vi "VgSweep_Bdep.vi"(8 "Start sweeping":bool) -> ()   [LabVIEW 2015]
uses:
  <vilib>/Utility/file.llb/Read From Spreadsheet File (DBL).vi
panel:
  in  "B-table String":string
  in  "Time Stamp":timestamp
  in  "Stabilisation (min)":dbl=0.8 max=4.0 step=1.0
  in  "Custom Folder":string
  out "Communication":string
  in  "Step (T)":dbl=12.0 min=-4.0 max=4.0 step=0.1 format="%.3f"
  out "Experiment ends at:":string
  out "B Array":dbl[](array[numeric])
  in  "Faster":dbl=10.0
  in  "HigherRateBack?":bool
  out "Hours":dbl format="%.1f"
  out "Estimated time of experiment:":i16
  out "# of connections":i16=1 min=-4 max=4 step=1
  in  "Final B (T)":dbl=12.0 min=-4.0 max=4.0 step=0.1 format="%.3f"
  in  "Initial B (T)":dbl min=-4.0 max=4.0 step=0.1 format="%.3f"
  in  "V2:":dbl=1.0 min=-4.0 max=4.0 step=0.1 format="%.3f"
  in  "Sweep rate , V/min":dbl=0.6 min=0.0 max=1.0 step=0.01 format="%.4f"
  in  "V1:":dbl min=-4.0 max=4.0 step=0.1 format="%.3f"
  # "Define interval of gate voltage\nfor main Keithley 2400 (address 12):"
  # "Copy and paste  the \nvalues of B field here.\nIf this string is empty \nthe table is filled \nautomatically."
  # "Set temperatures at which sweeps\nare made"
  # "Go to Initial T?"
  # "min."
  # "="
  # "hours"
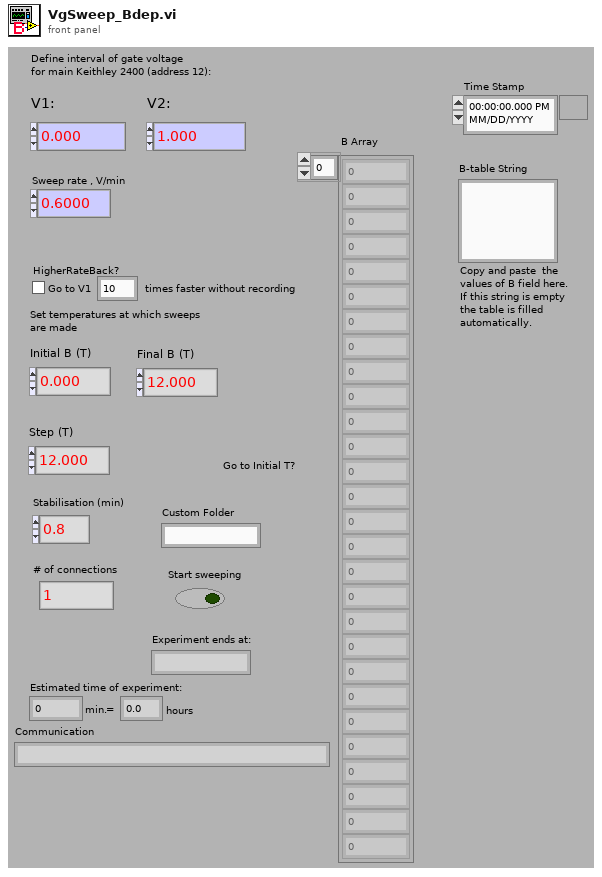
[diagram p1: front panel]
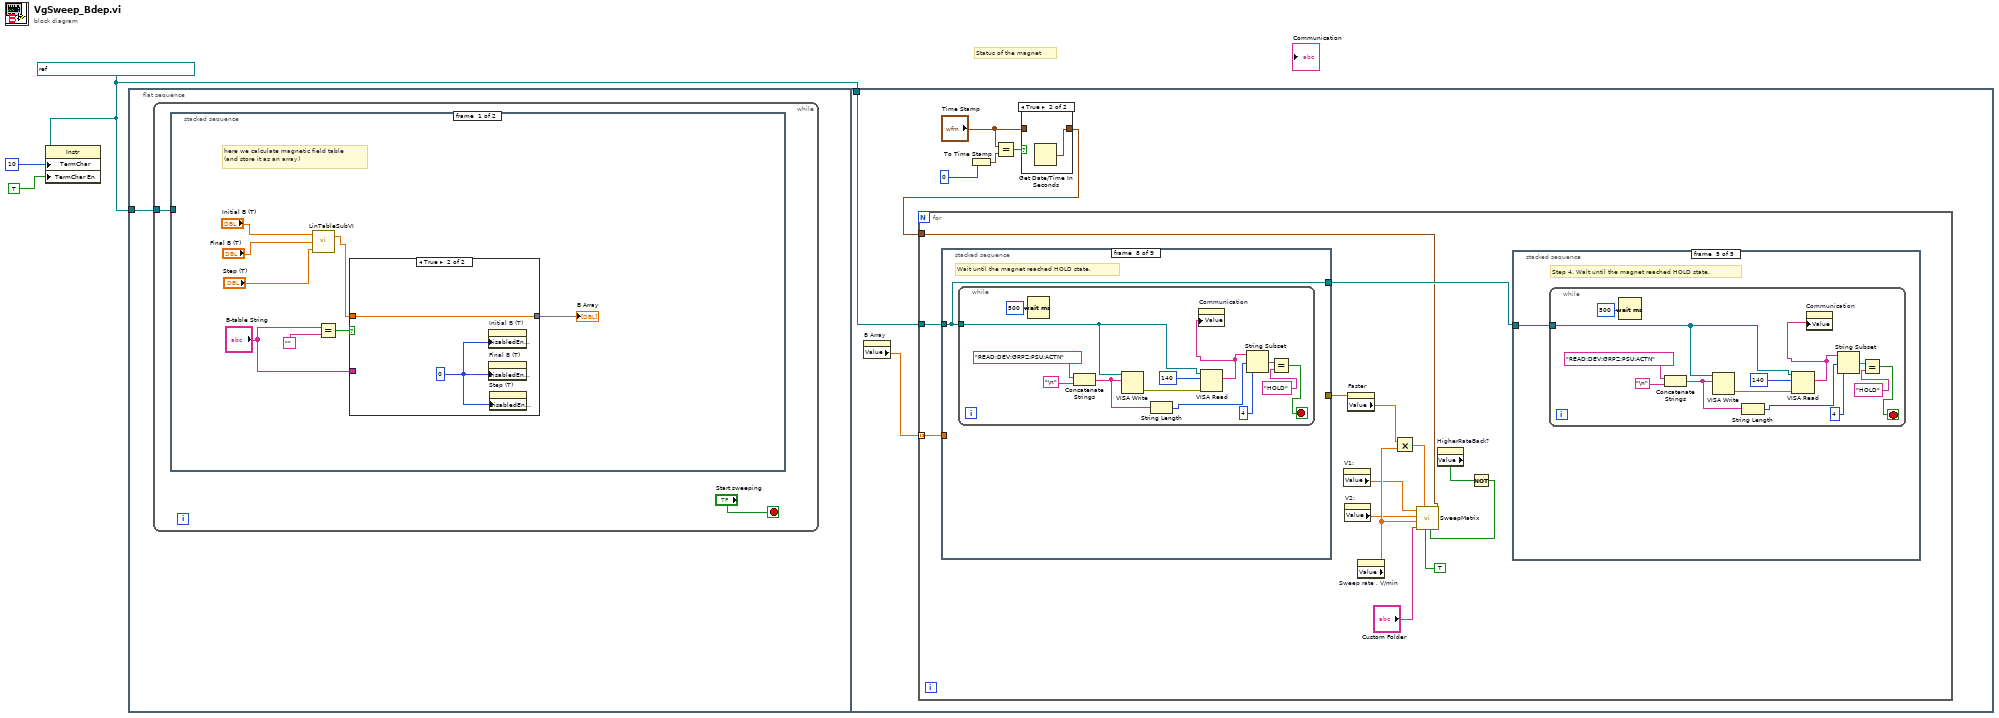
[diagram p0: block diagram]
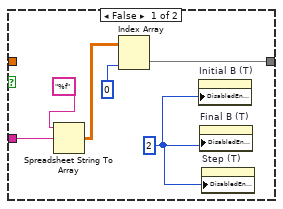
[diagram p2: hidden frame]
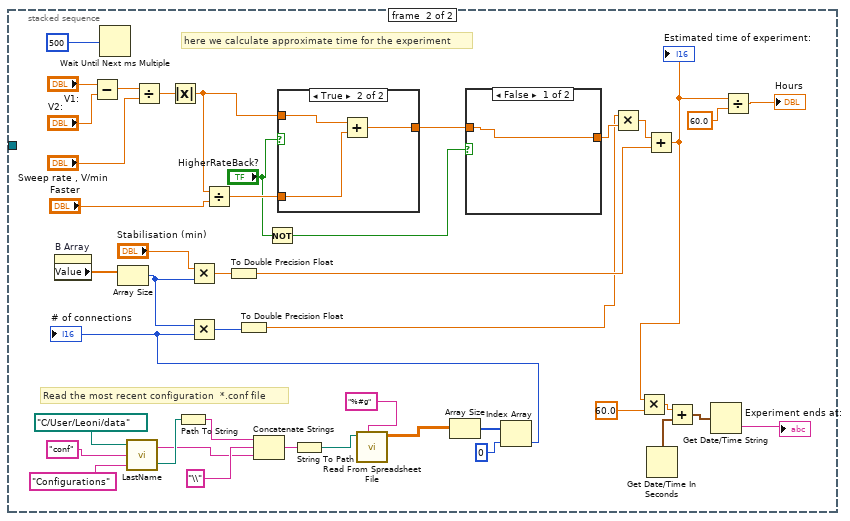
[diagram p3: hidden frame]
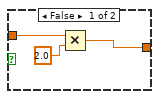
[diagram p4: hidden frame]
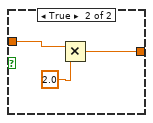
[diagram p5: hidden frame]
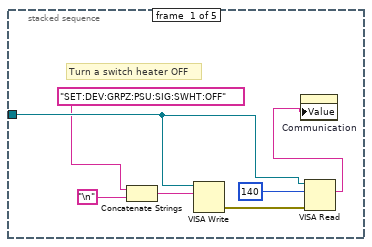
[diagram p7: hidden frame]
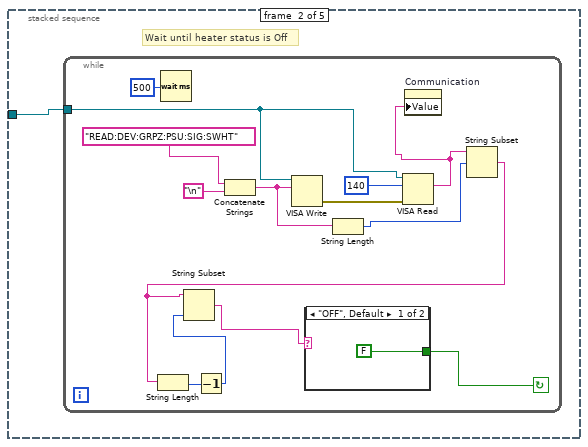
[diagram p8: hidden frame]
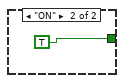
[diagram p9: hidden frame]
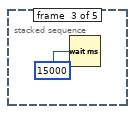
[diagram p10: hidden frame]
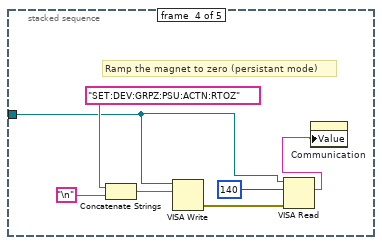
[diagram p11: hidden frame]
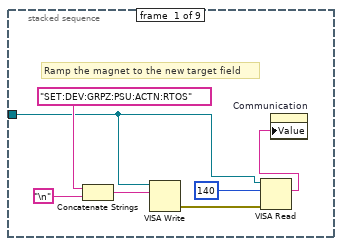
[diagram p12: hidden frame]
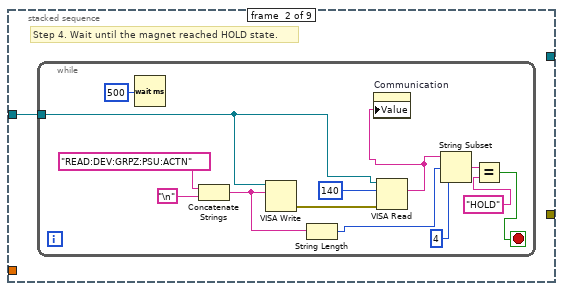
[diagram p13: hidden frame]
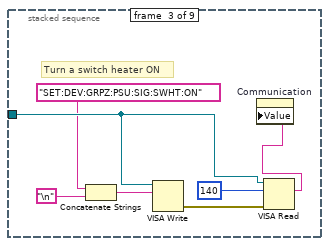
[diagram p14: hidden frame]
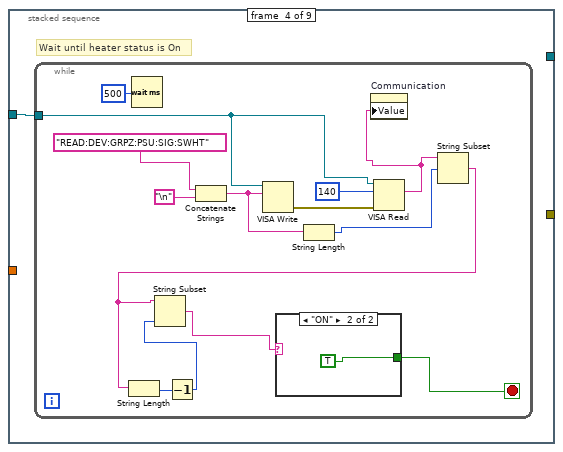
[diagram p15: hidden frame]
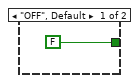
[diagram p16: hidden frame]
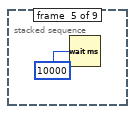
[diagram p17: hidden frame]
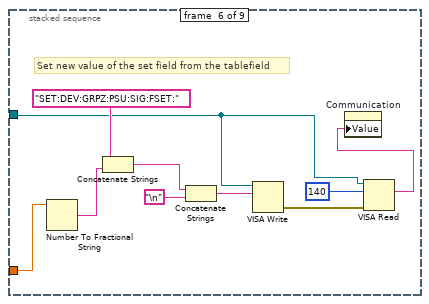
[diagram p18: hidden frame]
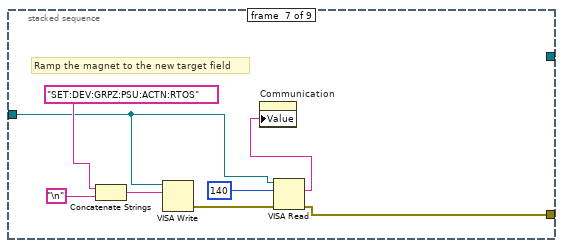
[diagram p19: hidden frame]
diagram:
  w1 = refnum<visa-resource-name> "TCPIP0::192.168.128.3::7020::SOCKET" ("VISA resource name")
  # "Status of the magnet"
  n1 = property class="Instr"(reference=w1, "TermChar"=10, "TermChar En"=TRUE) -> ()  [unwired: 1 in, 2 out]
  n2 = flat-sequence {
    tunnel: w1 -> [w4]
    tunnel: w1 -> [w82]
    frame #0 {
      n3 = while {
        tunnel: w4 -> [w5]
        stop <- "Start sweeping" stop-if-true
        n4 = stacked-sequence {
          tunnel: w5 -> [_ _]
          frame #0 {
            # "here we calculate magnetic field table\n(and store it as an array)"
            n5 = call "LinTableSubVI.vi"("Step"="Step (T)", "Final"="Final B (T)", "Initial"="Initial B (T)") -> ("Array"=w10:dbl[])  [unwired: 1 in]
            n6 = Equal?(x="B-table String", y="") -> (x = y?=w7:bool)
            n7 = case shown="True" w7 {
              tunnel: [w17 w22] -> w11
              tunnel: w10 -> [_ w22]
              tunnel: "B-table String" -> [w16 _]
              frame False {
                w15 = 2
                n8 = Spreadsheet String To Array(format string="%f", spreadsheet string=w16) -> (array=w19:dbl[][])  [unwired: 2 in]
                n9 = Index Array(array=w19, index (col)=0) -> (element=w17:dbl[])  [unwired: 1 in]
                n10 = property on="Initial B (T)" class="DigNum (strict)"("DisabledEnum"=w15) -> ()  [unwired: 2 in, 2 out]
                n11 = property on="Final B (T)" class="DigNum (strict)"("DisabledEnum"=w15) -> ()  [unwired: 2 in, 2 out]
                n12 = property on="Step (T)" class="DigNum (strict)"("DisabledEnum"=w15) -> ()  [unwired: 2 in, 2 out]
              }
              frame True {
                w21 = 0
                n13 = property on="Initial B (T)" class="DigNum (strict)"("DisabledEnum"=w21) -> ()  [unwired: 2 in, 2 out]
                n14 = property on="Final B (T)" class="DigNum (strict)"("DisabledEnum"=w21) -> ()  [unwired: 2 in, 2 out]
                n15 = property on="Step (T)" class="DigNum (strict)"("DisabledEnum"=w21) -> ()  [unwired: 2 in, 2 out]
              }
            }
            "B Array" <- w11
          }
          frame #1 {
            # "Read the most recent configuration  *.conf file"
            # "here we calculate approximate time for the experiment"
            n16 = property on="B Array" class="Arr (strict)"() -> ("Value"=w52:dbl[])  [unwired: 2 in, 2 out]
            n17 = Subtract(x="V1:", y="V2:") -> (x-y=w65:dbl)
            n18 = Wait Until Next ms Multiple(millisecond multiple=500) -> ()  [unwired: 1 out]
            n19 = Array Size(array=w52) -> (size(s)=w23:i32)
            n20 = call "LastName.vi"("Custom Folder"="Configurations", "Extention"="conf", "User Data Folder"=path "C:/User/Leoni/data") -> ("created path"=w47:path, "String"=w46:string)
            n21 = Divide(x=w65, y="Sweep rate , V/min") -> (x/y=w64:dbl)
            n22 = Absolute Value(x=w64) -> (abs(x)=w30:dbl)
            n23 = Path To String(path=w47) -> (string=w51:string)
            n24 = Multiply(x="Stabilisation (min)", y=w23) -> (x*y=w35:dbl)
            n25 = Divide(x=w30, y="Faster") -> (x/y=w31:dbl)
            n26 = To Double Precision Float(number=w35) -> (double precision float=w34:dbl)
            n27 = Concatenate Strings(w51, "\\", w46) -> (w49:string)
            n28 = Not(x="HigherRateBack?") -> (.not. x?=w24:bool)
            n29 = case shown="True" "HigherRateBack?" {
              tunnel: [w66 w71] -> w32
              tunnel: w31 -> [_ w70]
              tunnel: w30 -> [w67 w69]
              frame False {
                n30 = Multiply(x=w67, y=2.0) -> (x*y=w66:dbl)
              }
              frame True {
                n31 = Add(x=w69, y=w70) -> (x+y=w71:dbl)
              }
            }
            n32 = String To Path(string=w49) -> (path=w42:path)
            n33 = call-poly <vilib>:"Read From Spreadsheet File.vi"("format (%.3f)"="%#g", "file path (dialog if empty)"=w42) -> ("all rows"=w39:dbl[][])  [unwired: 5 in, 4 out]
            n34 = Array Size(array=w39) -> (size(s)=w41:i32[])
            n35 = case shown="False" w24 {
              tunnel: w32 -> [w72 w74]
              tunnel: [w72 w73] -> w29
              frame False {
              }
              frame True {
                n36 = Multiply(x=w74, y=2.0) -> (x*y=w73:dbl)
              }
            }
            n37 = Index Array(array=w41, index=0) -> (element=w38:i32)
            "# of connections" <- w38
            n38 = Multiply(x=w23, y=w38) -> (x*y=w27:i32)
            n39 = To Double Precision Float(number=w27) -> (double precision float=w26:dbl)
            n40 = Multiply(x=w26, y=w29) -> (x*y=w28:dbl)
            n41 = Add(x=w28, y=w34) -> (x+y=w36:dbl)
            "Estimated time of experiment:" <- w36
            n42 = Multiply(x=w36, y=60.0) -> (x*y=w56:dbl)
            n43 = Get Date/Time In Seconds() -> (seconds since 1Jan1904=w55:timestamp)
            n44 = Add(x=w56, y=w55) -> (x+y=w54:timestamp)
            n45 = Get Date/Time String(seconds (now)=w54) -> (time string=→"Experiment ends at:":string)  [unwired: 2 in, 1 out]
            n46 = Divide(x=w36, y=60.0) -> (x/y=→"Hours":dbl)
          }
        }
      }
    }
    frame #1 {
      n47 = property on="B Array" class="Arr (strict)"() -> ("Value"=w81:dbl[])  [unwired: 2 in, 2 out]
      n48 = To Time Stamp(1:0) -> (0:w79:timestamp)
      n49 = Equal?(x="Time Stamp", y=w79) -> (x = y?=w78:bool)
      n50 = case shown="True" w78 {
        tunnel: "Time Stamp" -> [w83 _]
        tunnel: [w83 w84] -> w76
        frame False {
        }
        frame True {
          n51 = Get Date/Time In Seconds() -> (seconds since 1Jan1904=w84:timestamp)
        }
      }
      n52 = for {
        tunnel: w82 -> [w98]
        tunnel: w81 -> [w97] mode=indexing
        tunnel: w76 -> [w85]
        n53 = stacked-sequence {
          tunnel: w98 -> [w145 w152 w167 w173 _ w193 w202 w209 _]
          tunnel: w97 -> [_ _ _ _ _ w192 _ _ _]
          tunnel: [_ _ _ _ _ _ _ w209 _] -> w87
          tunnel: [_ _ _ _ _ _ w201 _ _] -> w86
          frame #0 {
            # "Ramp the magnet to the new target field"
            n54 = Concatenate Strings("SET:DEV:GRPZ:PSU:ACTN:RTOS" ("string"), "\n") -> (w148:string)
            n55 = VISA Write(VISA resource name=w145, write buffer=w148) -> (error out=w151:errorcluster)  [unwired: 1 in, 2 out]
            n56 = VISA Read(VISA resource name=w145, byte count=140, error in (no error)=w151) -> (read buffer=w146:string)  [unwired: 3 out]
            n57 = property on="Communication" class="Str"("Value"=w146) -> ()  [unwired: 2 in, 2 out]
          }
          frame #1 {
            # "Step 4. Wait until the magnet reached HOLD state."
            n58 = while {
              tunnel: w152 -> [w162]
              stop <- w155 stop-if-true
              n59 = Wait (ms)(milliseconds to wait=500) -> ()  [unwired: 1 out]
              n60 = Concatenate Strings("READ:DEV:GRPZ:PSU:ACTN" ("string"), "\n") -> (w159:string)
              n61 = VISA Write(VISA resource name=w162, write buffer=w159) -> (error out=w165:errorcluster)  [unwired: 1 in, 2 out]
              n62 = String Length(string=w159) -> (length=w158:i32)
              n63 = VISA Read(VISA resource name=w162, byte count=140, error in (no error)=w165) -> (read buffer=w153:string)  [unwired: 3 out]
              n64 = property on="Communication" class="Str"("Value"=w153) -> ()  [unwired: 2 in, 2 out]
              n65 = String Subset(string=w153, offset (0)=w158, length (rest)=4) -> (substring=w157:string)
              n66 = Equal?(x=w157, y="HOLD") -> (x = y?=w155:bool)
            }
          }
          frame #2 {
            # "Turn a switch heater ON"
            n67 = Concatenate Strings("SET:DEV:GRPZ:PSU:SIG:SWHT:ON" ("string"), "\n") -> (w169:string)
            n68 = VISA Write(VISA resource name=w167, write buffer=w169) -> (error out=w172:errorcluster)  [unwired: 1 in, 2 out]
            n69 = VISA Read(VISA resource name=w167, byte count=140, error in (no error)=w172) -> (read buffer=w168:string)  [unwired: 3 out]
            n70 = property on="Communication" class="Str"("Value"=w168) -> ()  [unwired: 2 in, 2 out]
          }
          frame #3 {
            # "Wait until heater status is On"
            n71 = while {
              tunnel: w173 -> [w184]
              stop <- w175 stop-if-true
              n72 = Wait (ms)(milliseconds to wait=500) -> ()  [unwired: 1 out]
              n73 = Concatenate Strings("READ:DEV:GRPZ:PSU:SIG:SWHT" ("string"), "\n") -> (w183:string)
              n74 = VISA Write(VISA resource name=w184, write buffer=w183) -> (error out=w187:errorcluster)  [unwired: 1 in, 2 out]
              n75 = String Length(string=w183) -> (length=w182:i32)
              n76 = VISA Read(VISA resource name=w184, byte count=140, error in (no error)=w187) -> (read buffer=w180:string)  [unwired: 3 out]
              n77 = property on="Communication" class="Str"("Value"=w180) -> ()  [unwired: 2 in, 2 out]
              n78 = String Subset(string=w180, offset (0)=w182) -> (substring=w174:string)  [unwired: 1 in]
              n79 = String Length(string=w174) -> (length=w178:i32)
              n80 = Decrement(x=w178) -> (x-1=w177:i32)
              n81 = String Subset(string=w174, length (rest)=w177) -> (substring=w176:string)  [unwired: 1 in]
              n82 = case shown="\"ON\"" w176 {
                tunnel: [FALSE TRUE] -> w175
                frame "OFF", Default {
                }
                frame "ON" {
                }
              }
            }
          }
          frame #4 {
            n83 = Wait (ms)(milliseconds to wait=10000) -> ()  [unwired: 1 out]
          }
          frame #5 {
            # "Set new value of the set field from the tablefield"
            n84 = Number To Fractional String(number=w192) -> (F-format string=w199:string)  [unwired: 3 in]
            n85 = Concatenate Strings("SET:DEV:GRPZ:PSU:SIG:FSET:" ("string"), w199) -> (w194:string)
            n86 = Concatenate Strings(w194, "\n") -> (w195:string)
            n87 = VISA Write(VISA resource name=w193, write buffer=w195) -> (error out=w198:errorcluster)  [unwired: 1 in, 2 out]
            n88 = VISA Read(VISA resource name=w193, byte count=140, error in (no error)=w198) -> (read buffer=w191:string)  [unwired: 3 out]
            n89 = property on="Communication" class="Str"("Value"=w191) -> ()  [unwired: 2 in, 2 out]
          }
          frame #6 {
            # "Ramp the magnet to the new target field"
            n90 = Concatenate Strings("SET:DEV:GRPZ:PSU:ACTN:RTOS" ("string"), "\n") -> (w205:string)
            n91 = VISA Write(VISA resource name=w202, write buffer=w205) -> (error out=w208:errorcluster)  [unwired: 1 in, 2 out]
            n92 = VISA Read(VISA resource name=w202, byte count=140, error in (no error)=w208) -> (read buffer=w203:string, error out=w201:errorcluster)  [unwired: 2 out]
            n93 = property on="Communication" class="Str"("Value"=w203) -> ()  [unwired: 2 in, 2 out]
          }
          frame #7 {
            # "Wait until the magnet reached HOLD state."
            n94 = while {
              tunnel: w209 -> [w219]
              stop <- w212 stop-if-true
              n95 = Wait (ms)(milliseconds to wait=500) -> ()  [unwired: 1 out]
              n96 = Concatenate Strings("READ:DEV:GRPZ:PSU:ACTN" ("string"), "\n") -> (w216:string)
              n97 = VISA Write(VISA resource name=w219, write buffer=w216) -> (error out=w222:errorcluster)  [unwired: 1 in, 2 out]
              n98 = String Length(string=w216) -> (length=w215:i32)
              n99 = VISA Read(VISA resource name=w219, byte count=140, error in (no error)=w222) -> (read buffer=w210:string)  [unwired: 3 out]
              n100 = property on="Communication" class="Str"("Value"=w210) -> ()  [unwired: 2 in, 2 out]
              n101 = String Subset(string=w210, offset (0)=w215, length (rest)=4) -> (substring=w214:string)
              n102 = Equal?(x=w214, y="HOLD") -> (x = y?=w212:bool)
            }
          }
          frame #8 {
          }
        }
        n103 = property on="V1:" class="DigNum (strict)"() -> ("Value"=w90:dbl)  [unwired: 2 in, 2 out]
        n104 = property on="V2:" class="DigNum (strict)"() -> ("Value"=w89:dbl)  [unwired: 2 in, 2 out]
        n105 = property on="Faster" class="DigNum (strict)"(error in=w86) -> ("Value"=w93:dbl)  [unwired: 1 in, 2 out]
        n106 = property on="Sweep rate , V/min" class="DigNum (strict)"() -> ("Value"=w94:dbl)  [unwired: 2 in, 2 out]
        n107 = Multiply(x=w93, y=w94) -> (x*y=w95:dbl)
        n108 = property on="HigherRateBack?" class="Bool (strict)"() -> ("Value"=w92:bool)  [unwired: 2 in, 2 out]
        n109 = Not(x=w92) -> (.not. x?=w96:bool)
        n110 = call "SweepMatrix.vi"("Time Stamp"=w85, "From V2 to V1"=w96, "Play Button"=TRUE, "Rate w/o measure, V/min"=w95, "Custom Folder"="Custom Folder", "Sweep rate, V/min"=w94, "V2 (V)"=w89, "V1 (V)"=w90) -> ()  [unwired: 4 in]
        n111 = stacked-sequence {
          tunnel: w87 -> [w101 w106 _ w125 w131]
          frame #0 {
            # "Turn a switch heater OFF"
            n112 = Concatenate Strings("SET:DEV:GRPZ:PSU:SIG:SWHT:OFF" ("string"), "\n") -> (w102:string)
            n113 = VISA Write(VISA resource name=w101, write buffer=w102) -> (error out=w105:errorcluster)  [unwired: 1 in, 2 out]
            n114 = VISA Read(VISA resource name=w101, byte count=140, error in (no error)=w105) -> (read buffer=w99:string)  [unwired: 3 out]
            n115 = property on="Communication" class="Str"("Value"=w99) -> ()  [unwired: 2 in, 2 out]
          }
          frame #1 {
            # "Wait until heater status is Off"
            n116 = while {
              tunnel: w106 -> [w117]
              stop <- w109 continue-if-true
              n117 = Wait (ms)(milliseconds to wait=500) -> ()  [unwired: 1 out]
              n118 = Concatenate Strings("READ:DEV:GRPZ:PSU:SIG:SWHT" ("string"), "\n") -> (w116:string)
              n119 = VISA Write(VISA resource name=w117, write buffer=w116) -> (error out=w120:errorcluster)  [unwired: 1 in, 2 out]
              n120 = String Length(string=w116) -> (length=w115:i32)
              n121 = VISA Read(VISA resource name=w117, byte count=140, error in (no error)=w120) -> (read buffer=w107:string)  [unwired: 3 out]
              n122 = property on="Communication" class="Str"("Value"=w107) -> ()  [unwired: 2 in, 2 out]
              n123 = String Subset(string=w107, offset (0)=w115) -> (substring=w108:string)  [unwired: 1 in]
              n124 = String Length(string=w108) -> (length=w112:i32)
              n125 = Decrement(x=w112) -> (x-1=w111:i32)
              n126 = String Subset(string=w108, length (rest)=w111) -> (substring=w110:string)  [unwired: 1 in]
              n127 = case shown="\"OFF\", Default" w110 {
                tunnel: [FALSE TRUE] -> w109
                frame "OFF", Default {
                }
                frame "ON" {
                }
              }
            }
          }
          frame #2 {
            n128 = Wait (ms)(milliseconds to wait=15000) -> ()  [unwired: 1 out]
          }
          frame #3 {
            # "Ramp the magnet to zero (persistant mode)"
            n129 = Concatenate Strings("SET:DEV:GRPZ:PSU:ACTN:RTOZ" ("string"), "\n") -> (w127:string)
            n130 = VISA Write(VISA resource name=w125, write buffer=w127) -> (error out=w130:errorcluster)  [unwired: 1 in, 2 out]
            n131 = VISA Read(VISA resource name=w125, byte count=140, error in (no error)=w130) -> (read buffer=w124:string)  [unwired: 3 out]
            n132 = property on="Communication" class="Str"("Value"=w124) -> ()  [unwired: 2 in, 2 out]
          }
          frame #4 {
            # "Step 4. Wait until the magnet reached HOLD state."
            n133 = while {
              tunnel: w131 -> [w141]
              stop <- w134 stop-if-true
              n134 = Wait (ms)(milliseconds to wait=500) -> ()  [unwired: 1 out]
              n135 = Concatenate Strings("READ:DEV:GRPZ:PSU:ACTN" ("string"), "\n") -> (w138:string)
              n136 = VISA Write(VISA resource name=w141, write buffer=w138) -> (error out=w144:errorcluster)  [unwired: 1 in, 2 out]
              n137 = String Length(string=w138) -> (length=w137:i32)
              n138 = VISA Read(VISA resource name=w141, byte count=140, error in (no error)=w144) -> (read buffer=w132:string)  [unwired: 3 out]
              n139 = property on="Communication" class="Str"("Value"=w132) -> ()  [unwired: 2 in, 2 out]
              n140 = String Subset(string=w132, offset (0)=w137, length (rest)=4) -> (substring=w136:string)
              n141 = Equal?(x=w136, y="HOLD") -> (x = y?=w134:bool)
            }
          }
        }
      }
    }
  }
